vi "Limit Switches.vi"(1 "Desired Motion":dbl, 2 "Lower Bound":dbl, 3 "Input":dbl, 4 "Upper Bound":dbl) -> (0 "Allowed Motion":dbl)   [LabVIEW 2015]
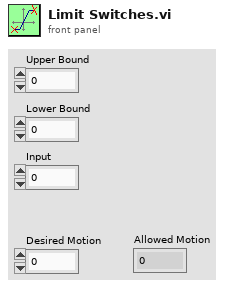
[diagram p1: front panel]
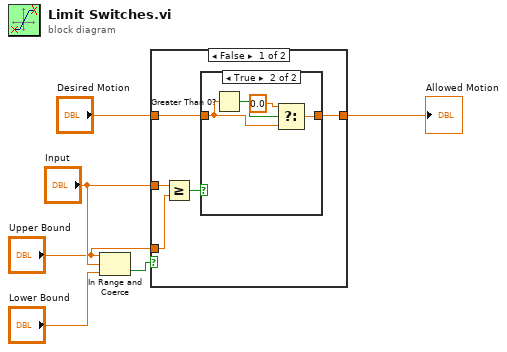
[diagram p0: block diagram]
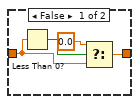
[diagram p2: hidden frame]
diagram:
  n1 = In Range and Coerce(upper limit="Upper Bound", x="Input", lower limit="Lower Bound") -> (In Range?=w5:bool)  [unwired: 1 out]
  n2 = case shown="False" w5 {
    tunnel: "Input" -> [w11 _]
    tunnel: "Upper Bound" -> [w10 _]
    tunnel: "Desired Motion" -> [w8 w20]
    tunnel: [w7 w20] -> w1
    frame False {
      n3 = Greater Or Equal?(x=w11, y=w10) -> (x >= y?=w9:bool)
      n4 = case shown="True" w9 {
        tunnel: w8 -> [w14 w17]
        tunnel: [w12 w16] -> w7
        frame False {
          n5 = Less Than 0?(x=w14) -> (x < 0?=w15:bool)
          n6 = Select(t=0.0, s=w15, f=w14) -> (s? t:f=w12:dbl)
        }
        frame True {
          n7 = Greater Than 0?(x=w17) -> (x > 0?=w19:bool)
          n8 = Select(t=0.0, s=w19, f=w17) -> (s? t:f=w16:dbl)
        }
      }
    }
    frame True {
    }
  }
  "Allowed Motion" <- w1
